vi "Update Log Path box colors.vi"(9 "Force Default Colors? (F)":bool, 10 "Path Refnum in":refnum<vi>, 11 "Settings in":T1) -> (3 "Settings out":T1)   [LabVIEW 2021, in "Settings.lvlib"]
doc: "Change the colors of the file path text box according to whether the data log file be overwritten: default colors when safe, red tint when overwriting."
uses:
  Settings.lvlib
  Settings.ctl
  Acquisition/Hardware Configuration.ctl
  Acquisition/Channel Settings.ctl
  Acquisition/IO Device.ctl
  Interval Timer/Repeat Interval.ctl
  Interval Timer/Interval Length.ctl
  Interval Timer/Interval Token.ctl
  Logging/Logging Configuration.ctl
  Diagnostics/Diagnostics Configuration.ctl
  <vilib>/Utility/miscctls.llb/LVTextColorsTypeDef.ctl
  Acquisition/Acquisition.lvlib
  Interval Timer/Interval Timer.lvlib
  Logging/Logging.lvlib
  Diagnostics/Diagnostics.lvlib
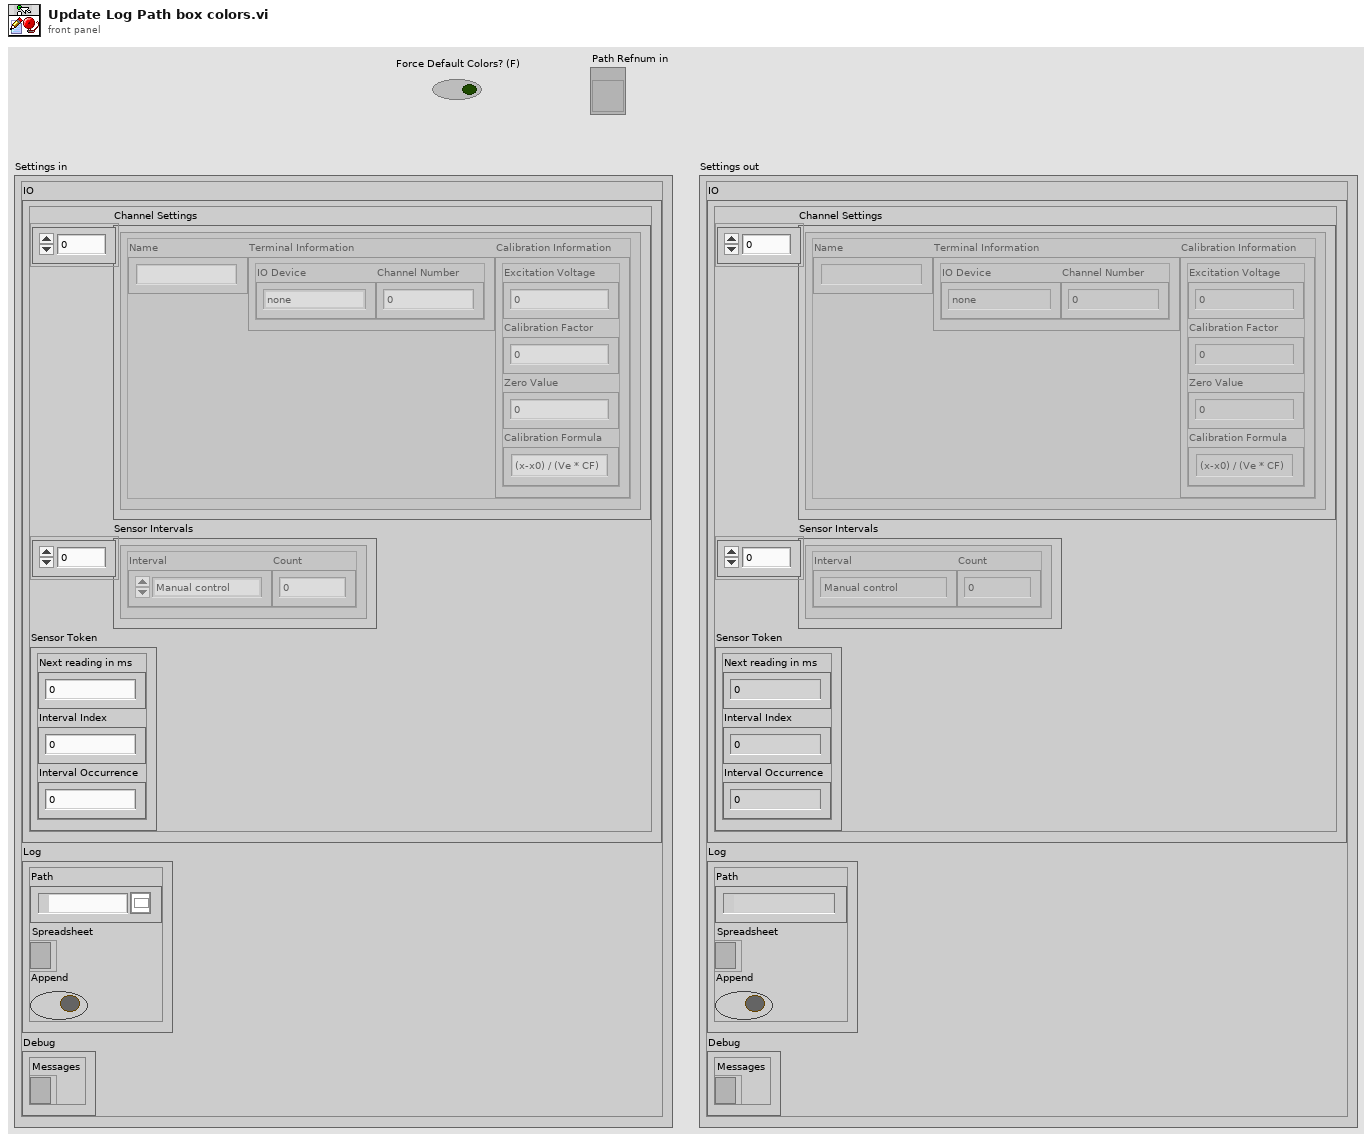
[diagram p1: front panel]
types:
  T1 = typedef "Settings.lvlib/Settings.ctl" = cluster{"IO":T2, "Log":T8, "Debug":T9}
  T2 = typedef "Acquisition.lvlib/Hardware Configuration.ctl" = cluster{"Channel Settings":T3[], "Sensor Intervals":T5[], "Sensor Token":T7}
  T3 = typedef "Acquisition.lvlib/Channel Settings.ctl" = cluster{"Name":string, "Terminal Information":cluster{"IO Device":T4, "Channel Number":i32}, "Calibration Information":cluster{"Excitation Voltage":dbl, "Calibration Factor":dbl, "Zero Value":dbl, "Calibration Formula":string}}
  T4 = typedef "Acquisition.lvlib/IO Device.ctl" = enum16{"none", "9219", "9401"}
  T5 = typedef "Interval Timer.lvlib/Repeat Interval.ctl" = cluster{"Interval":T6, "Count":i32}
  T6 = typedef "Interval Timer.lvlib/Interval Length.ctl" = enum16{"Manual control", "1 second", "10 seconds", "30 seconds", "60 seconds", "600 seconds", "1200 seconds", "3600 seconds"}
  T7 = typedef "Interval Timer.lvlib/Interval Token.ctl" = cluster{"Next reading in ms":u32, "Interval Index":i32, "Interval Occurrence":i32}
  T8 = typedef "Logging.lvlib/Logging Configuration.ctl" = cluster{"Path":path, "Spreadsheet":refnum<file>, "Append":bool}
  T9 = typedef "Diagnostics.lvlib/Diagnostics Configuration.ctl" = cluster{"Messages":refnum<file>}
  T10 = typedef "LVTextColorsTypeDef.ctl" = cluster{"Text Color":u32, "Background Color":u32}
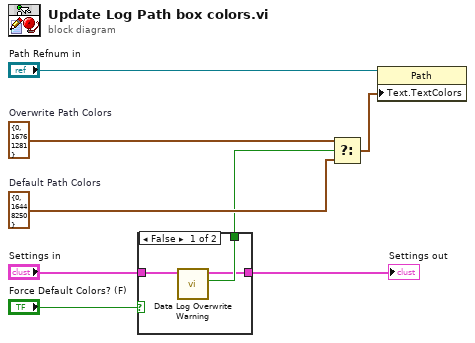
[diagram p0: block diagram]
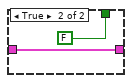
[diagram p2: hidden frame]
diagram:
  w6 = T10 {"Text Color"=0, "Background Color"=16448250}  # Default Path Colors
  w7 = T10 {"Text Color"=0, "Background Color"=16761281}  # Overwrite Path Colors
  n1 = case shown="False" "Force Default Colors? (F)" {
    tunnel: [w11 FALSE ("Overwrite Warning?")] -> w5
    tunnel: [w10 w13] -> w4
    tunnel: "Settings in" -> [w9 w13]
    frame False {
      n2 = call "Data Log Overwrite Warning.vi"("Settings in"=w9) -> ("Overwrite Warning?"=w11:bool, "Settings out"=w10:T1)  [unwired: 8 in, 1 out]
    }
    frame True {
    }
  }
  "Settings out" <- w4
  n3 = Select(t=w7, s=w5, f=w6) -> (s? t:f=w8:T10)
  n4 = property on="Property Node" class="Path"(reference="Path Refnum in", "Text.TextColors"=w8) -> ()  [unwired: 1 in, 2 out]
